vi "RunExecutable.vi"() -> ()   [LabVIEW 2013]
doc: "Sample VI that shows how to run an executable with optional inputs from inside LabVIEW\n\nYou must tell LabVIEW the location of the executable\n\nYou must tell LabVIEW what directory you are working in\n\nR. Sheehan 6 - 12 - 2018"
panel:
  out "return code":i32
  in  "wait until completion? (T)":bool=TRUE
  out "standard error":string
  out "standard output":string
  in  "working directory":path=path ""
  in  "command line":string
  # "It should be a simple enough matter to have the file names as inputs\n\nYou could also implement an error cluster that will run or otherwise\ndepending on the inputs"
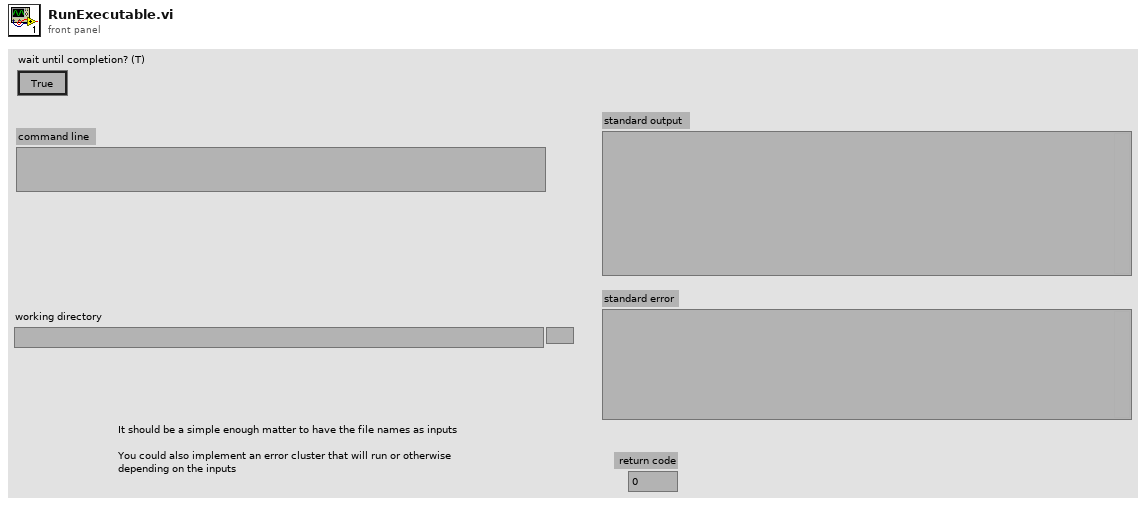
[diagram p1: front panel]
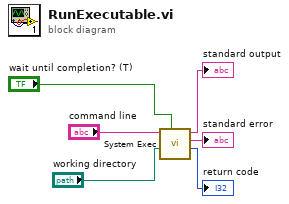
[diagram p0: block diagram]
diagram:
  n1 = call <vilib>:"System Exec.vi"("wait until completion? (T)"="wait until completion? (T)", "working directory"="working directory", "command line"="command line") -> ("return code"=→"return code":i32, "standard error"=→"standard error":string, "standard output"=→"standard output":string)  [unwired: 5 in, 1 out]
